vi "Robot Global Data.vi"() -> ()   [LabVIEW 2015]
doc: "This global VI can contain as many global variables as you need. Place a control on the panel, give it a good name. To read or write to it from a VI, drag the icon to the diagram of that VI. You can also drag from the project. Click on the node to change which global you access. You shouldn't have multiple locations writing to a global or it will cause a race-condition."
uses:
  <vilib>/Rock Robotics/WPI/Camera/WPI_CameraImageSize.ctl
  <vilib>/Rock Robotics/WPI/DriverStation/WPI_DriverStationRobotMode2.ctl
panel:
  in  "Joystick Butt 18":bool
  in  "Joystick Butt 17":bool
  in  "Joystick Butt 16":bool
  in  "Joystick Butt 15":bool
  in  "Joystick Butt 14":bool
  in  "Joystick Butt 13":bool
  in  "Joystick Throttle":dbl(slide) scale=0.0..10.0
  in  "Joystick Y":dbl(slide) scale=0.0..10.0
  in  "Joystick X":dbl(slide) scale=0.0..10.0
  in  "Joystick Butt 12":bool
  in  "Joystick Butt 11":bool
  in  "Joystick Butt 10":bool
  in  "Joystick Butt 9":bool
  in  "Joystick Butt 8":bool
  in  "Joystick Butt 7":bool
  in  "Joystick Butt 6":bool
  in  "Joystick Butt 5":bool
  in  "Joystick Butt 4":bool
  in  "Joystick Butt 3":bool
  in  "Joystick Butt 2":bool
  in  "Joystick Butt 1":bool
  in  "Auto Butt 12":bool
  in  "Auto Butt 11":bool
  in  "Auto Butt 10":bool
  in  "Auto Butt 9":bool
  in  "Auto Butt 8":bool
  in  "Auto Butt 7":bool
  in  "Auto Butt 6":bool
  in  "Auto Butt 5":bool
  in  "Auto Butt 4":bool
  in  "Auto Butt 3":bool
  in  "Auto Butt 2":bool
  in  "Auto Butt 1":bool
  in  "Drive Mode":bool
  in  "Target Distance":dbl
  in  "Target Y":dbl
  in  "Target X":dbl
  in  "Robot Mode":T1
  out "ms to process":u32
  out "Detected Totes":T2(array[cluster]) {"Normalized Rect"."Numeric 5" format="%#_2g"; "Normalized Rect"."Numeric 3" format="%#_2g"; "Normalized Rect"."Numeric 2" format="%#_2g"; "Normalized Rect"."Numeric" format="%#_2g"}
  in  "image size":T3=enum."320x240"
  in  "Enable Vision":bool
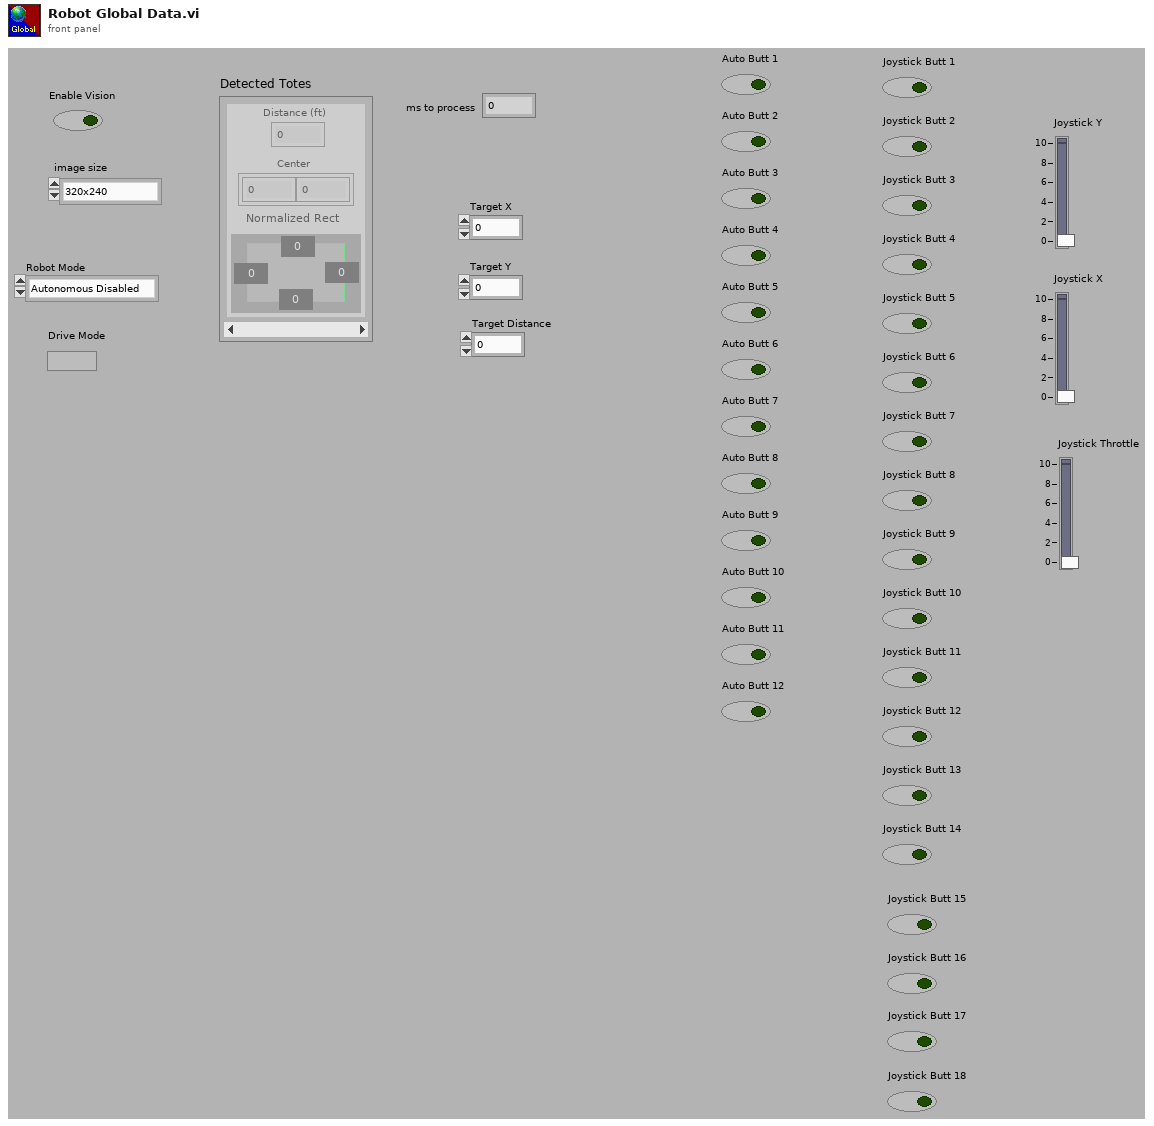
[diagram p1: front panel]
types:
  T1 = typedef "WPI_DriverStationRobotMode2.ctl" = enum16{"Autonomous Disabled", "Autonomous Enabled", "Teleop Disabled", "Teleop Enabled", "Disconnected", "Finish", "Test Disabled", "Test Enabled", "Emergency Stopped"}
  T2 = cluster{"Distance (ft)":dbl, "Center":cluster{dbl, dbl}, "Normalized Rect":cluster{"Numeric":dbl, "Numeric 2":dbl, "Numeric 3":dbl, "Numeric 5":dbl}}[]
  T3 = typedef "WPI_CameraImageSize.ctl" = enum16{"640x480", "320x240", "160x120", "Custom"}
diagram:
